vi "Set Shared Variable Refnum.vi"(8 "error in (no error)":errorcluster, 10 "shared variable refnum":refnum<k21>, 11 "abs_SharedVar_Bool in":refnum<class "abs_SharedVar_Bool.lvclass">) -> (0 "error out":errorcluster, 3 "abs_SharedVar_Bool out":refnum<class "abs_SharedVar_Bool.lvclass">)   [LabVIEW 2021, in "abs_SharedVar_Bool.lvclass"]
uses:
  abs_SharedVar_Bool.lvclass
  abs_SharedVar_Bool.lvclass/abs_SharedVar_Bool.ctl
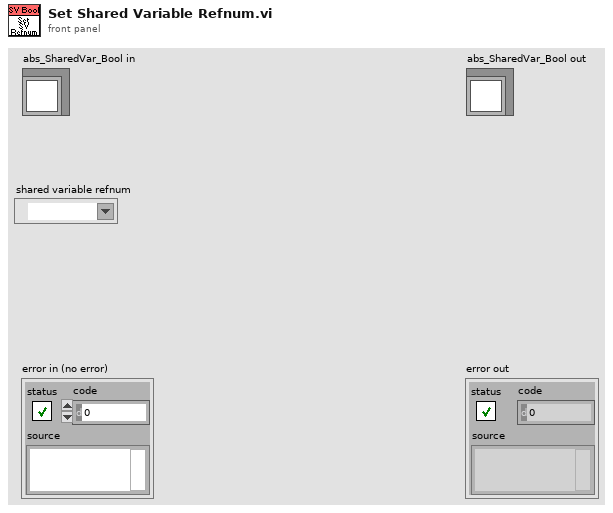
[diagram p1: front panel]
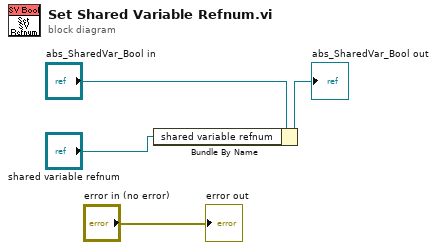
[diagram p0: block diagram]
diagram:
  n1 = Bundle By Name(cluster="abs_SharedVar_Bool in", "shared variable refnum"="shared variable refnum") -> (→"abs_SharedVar_Bool out":refnum<class "abs_SharedVar_Bool.lvclass">)
  "error out" <- "error in (no error)"
